vi "Sort Editors.vi"(10 "Panel B":refnum<class "Panel.lvclass">, 11 "Panel A":refnum<class "Panel.lvclass">) -> (3 "A < B":bool)   [LabVIEW 2020, in "FlexBlocks.lvlib"]
uses:
  FlexBlocks.lvlib
  <vilib>/IlluminatedG/IG OOPanel/OOPanel/Panel/Panel.lvclass
  Value Editor Base/Value Editor Base.lvclass
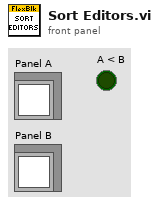
[diagram p1: front panel]
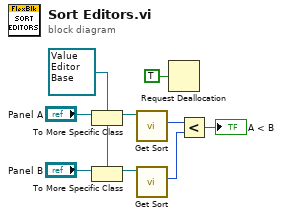
[diagram p0: block diagram]
diagram:
  w7 = refnum<class "Value Editor Base.lvclass"> refnum ("FlexBlocks.lvlib:Value Editor Base.lvclass")
  n1 = To More Specific Class(target class=w7, reference="Panel A") -> (specific class reference=w6:refnum<class "Value Editor Base.lvclass">)  [unwired: 1 in, 1 out]
  n2 = To More Specific Class(target class=w7, reference="Panel B") -> (specific class reference=w5:refnum<class "Value Editor Base.lvclass">)  [unwired: 1 in, 1 out]
  n3 = call "Get Sort.vi"("Value Editor Base in"=w6) -> ("Sort"=w4:i32)  [unwired: 8 in, 2 out]
  n4 = call "Get Sort.vi"("Value Editor Base in"=w5) -> ("Sort"=w3:i32)  [unwired: 8 in, 2 out]
  n5 = Request Deallocation(TRUE ("flag")) -> ()
  n6 = Less?(x=w4, y=w3) -> (x < y?=→"A < B":bool)
